vi "TrimOffTopBit.vi"(10 "8bitMnemonic in":string) -> (2 "7bitMnemonic":string)   [LabVIEW 2018]
panel:
  out "7bitValue":u8 format="%02x"
  out "7bits":bool[](array[boolean])
  out "8bits":bool[](array[boolean])
  out "8bitValue":u8 format="%02x"
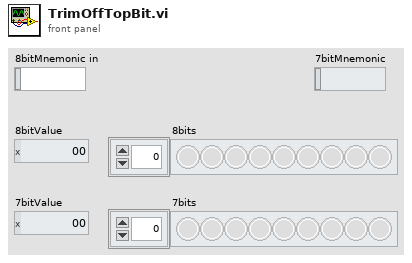
[diagram p1: front panel]
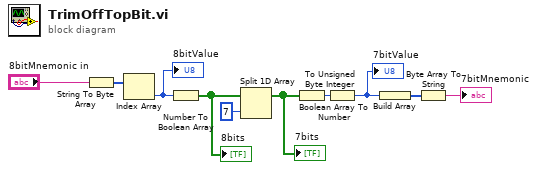
[diagram p0: block diagram]
diagram:
  n1 = String To Byte Array(string="8bitMnemonic in") -> (unsigned byte array=w6:u8[])
  n2 = Index Array(array=w6) -> (element=w7:u8)  [unwired: 1 in]
  "8bitValue" <- w7
  n3 = Number To Boolean Array(number=w7) -> (Boolean array=w3:bool[])
  "8bits" <- w3
  n4 = Split 1D Array(array=w3, index=7) -> (first subarray=w5:bool[])  [unwired: 1 out]
  "7bits" <- w5
  n5 = Boolean Array To Number(Boolean array=w5) -> (number=w8:u32)
  n6 = To Unsigned Byte Integer(number=w8) -> (unsigned 8bit integer=w1:u8)
  "7bitValue" <- w1
  n7 = Build Array(w1) -> (w2:u8[])
  n8 = Byte Array To String(unsigned byte array=w2) -> (string=→"7bitMnemonic":string)
